vi "Convolutions Tester.vi"() -> ()   [LabVIEW 2023]
uses:
  Images/_Images.ctl
  SubVIs/FLT/Conv Flt Presets.ctl
panel:
  out "Kernel":sgl[][](array[numeric])
  in  "Filter":T1=enum."Seifert 5x5"
  out "Image Src":T2(plugin-control)
  in  "Image":T3=enum."Connector1"
  in  "stop":bool
  out "Image Dst":T2(plugin-control)
  # "Simple Convolutions - Tester"
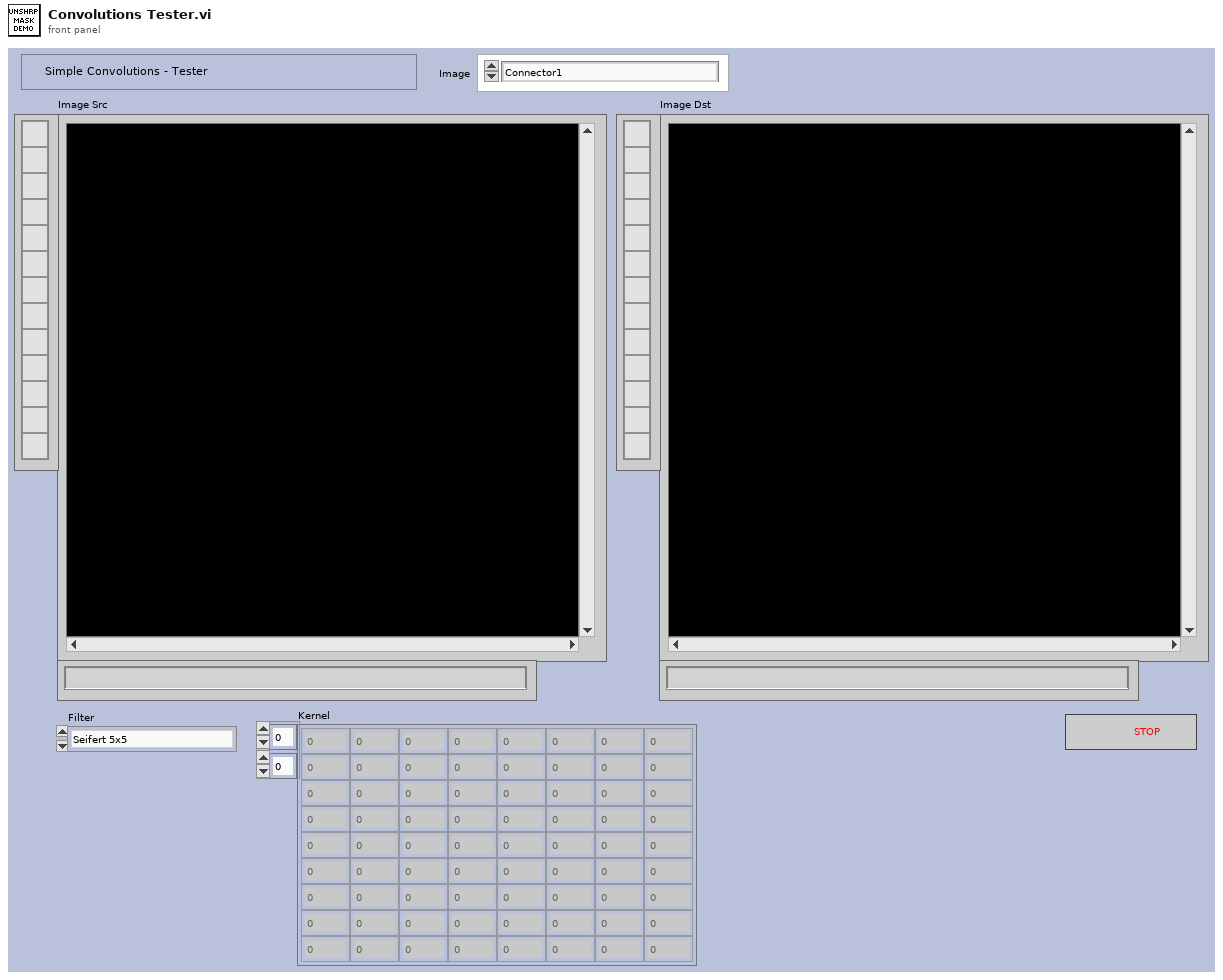
[diagram p1: front panel]
types:
  T1 = typedef "Conv Flt Presets.ctl" = enum16{"None", "Seifert 5x5", "Seifert 7x7", "High Pass 5x5 ", "High Pass 7x7", "Highlight Details 3x3", "Highlight Details 5x5", "Highlight Detail 7x7"}
  T2 = typedef "IMAQ Image.ctl" = refnum<image>
  T3 = typedef "_Images.ctl" = enum16{"Balls2", "Battery1", "Battery2", "Connector1", "Subwoofer1", "Subwoofer2", "Subwoofer3", "Subwoofer4", "Hase1", "Lamp1", "Lamp2", "Mouse1", "PhotoLens1", "Po1", "PowerSupply1", "Router", "--- Step Wedges ---", "Stepwedge1", "Stepwedge2", "Stepwedge3", "--- Fusion ---", "Fusion160kV", "Fusion2-120kV", "Fusion2-320kV", "Fusion300kV", "FusionPart1-120kV", "FusionPart1-180kV", "--- PART 01 ---", "Part1", "Part2", "Part3", "Part4", "Part5", "Part6", "Part7", "Part8", "--- Different Integrations ---", "Step2737-02Int", "Step2737-04Int", "Step2737-08Int", "Step2737-16Int", "Step2737-32Int", "Step2737-64Int"}
  T4 = typedef "Image Type" = u32
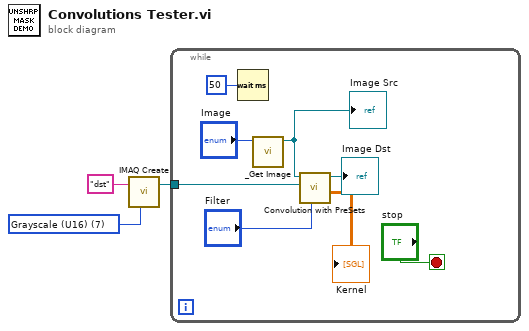
[diagram p0: block diagram]
diagram:
  w2 = T4 7 items=["Grayscale (U8)", "Grayscale (I16)", "Grayscale (SGL)", "Complex (CSG)", "RGB (U32)", "HSL (U32)", "RGB (U64)", "Grayscale (U16)"] ("Image Type")
  n1 = call "IMAQ Create"("Image Name"="dst", "Image Type"=w2) -> ("New Image"=w1:T2)  [unwired: 3 in, 1 out]
  n2 = while {
    tunnel: w1 -> [w7]
    stop <- "stop" stop-if-true
    n3 = Wait (ms)(milliseconds to wait=u32 50) -> ()  [unwired: 1 out]
    n4 = call "_Get Image.vi"("Image"="Image") -> ("Image Out"=w8:T2)  [unwired: 7 in, 3 out]
    "Image Src" <- w8
    n5 = call "Convolution with PreSets.vi"("Filter"="Filter", "Image Dst"=w7, "Image Src"=w8) -> ("Kernel"=→"Kernel":sgl[][], "Image Dst Out"=→"Image Dst":T2)  [unwired: 6 in, 1 out]
  }
